vi "Write Conveyors.vi"(8 "error in (no error)":errorcluster, 10 "Conveyors":refnum<class "ODESimulator_Base_Conveyor.lvclass">[](array[class]), 11 "ODESimulator_Base_Robot in":refnum<class "ODESimulator_Base_Robot.lvclass">) -> (0 "error out":errorcluster, 3 "ODESimulator_Base_Robot out":refnum<class "ODESimulator_Base_Robot.lvclass">)   [LabVIEW 2017, in "NI_Robotics_Simulator.lvlib" / "ODESimulator_Base_Robot.lvclass"]
uses:
  <vilib>/robotics/Simulator/Robot Classes/Base/ODESimulator_Base_Robot.lvclass
  <vilib>/robotics/Simulator/Robot Factory/Conveyor/Base/ODESimulator_Base_Conveyor.lvclass
  <vilib>/robotics/Simulator/Robot Classes/Base/ODESimulator_Base_Robot.lvclass/ODESimulator_Base_Robot.ctl
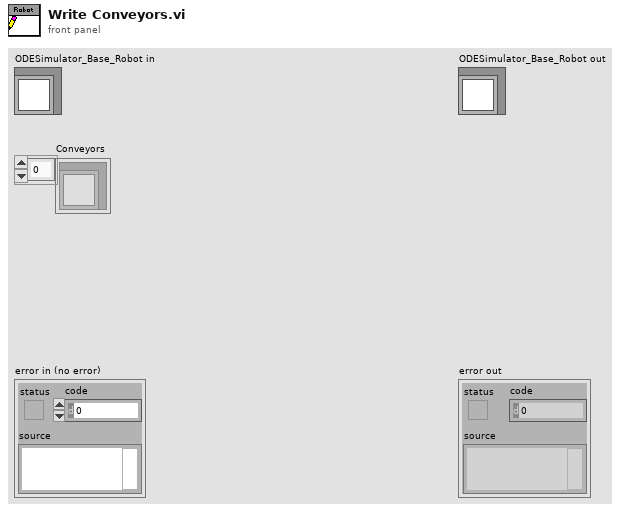
[diagram p1: front panel]
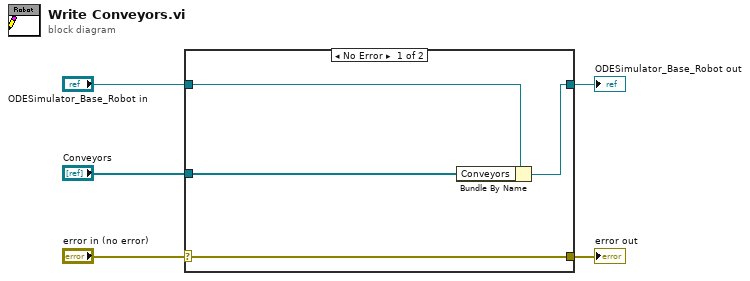
[diagram p0: block diagram]
diagram:
  n1 = case shown="No Error" "error in (no error)" {
    selector: "error in (no error)" -> [w9 w10]
    tunnel: [w9 w10] -> w4
    tunnel: [w7 w11] -> w2
    tunnel: "ODESimulator_Base_Robot in" -> [w8 w11]
    tunnel: "Conveyors" -> [w6 _]
    frame No Error {
      n2 = Bundle By Name(cluster=w8, "Conveyors"=w6) -> (w7:refnum<class "ODESimulator_Base_Robot.lvclass">)
    }
    frame Error {
    }
  }
  "error out" <- w4
  "ODESimulator_Base_Robot out" <- w2
